vi "Ball Carrying Logic.vi"(0 "Backwards Trigger":dbl, 1 "Had Ball Before?":bool, 3 "Rollers Active? in":bool, 4 "Safty Frist Angle":dbl, 5 "Warmup Initiation":bool, 6 "Fire from Load Delay":i32, 7 "Intake Angle":dbl, 10 "Angle in":dbl, 11 "Intake at Dangerous Height?":bool, 12 "Roll Backward Delay":u32, 13 "Ball Loaded? in":bool) -> (14 "Rollers Active? out":bool, 15 "Angle out":dbl, 17 "Trigger Out":dbl, 18 "Ball Loaded? out":bool)   [LabVIEW 2015]
uses:
  Common Code/Change Detect Boolean.vi
  <vilib>/Rock Robotics/WPI/DriverStation/WPI_DriverStationRobotMode2.ctl
panel:
  in  "Safty Frist?":bool
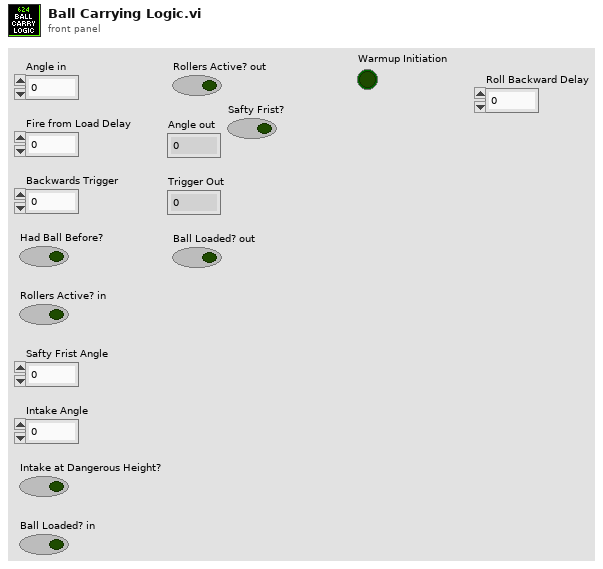
[diagram p1: front panel]
types:
  T1 = typedef "WPI_DriverStationRobotMode2.ctl" = enum16{"Autonomous Disabled", "Autonomous Enabled", "Teleop Disabled", "Teleop Enabled", "Disconnected", "Finish", "Test Disabled", "Test Enabled", "Emergency Stopped"}
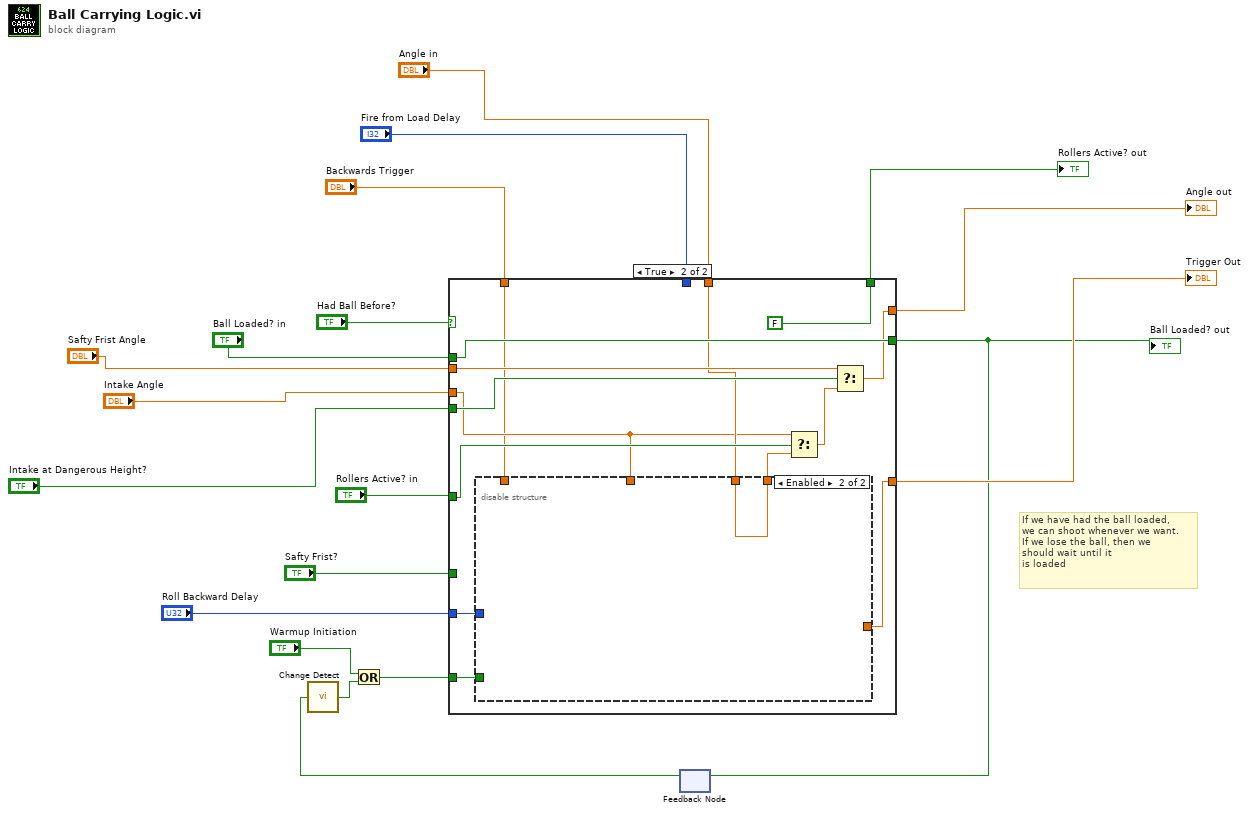
[diagram p0: block diagram]
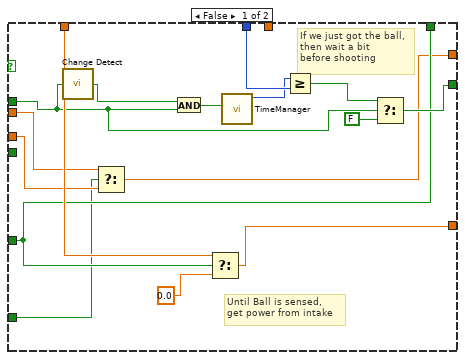
[diagram p2: hidden frame]
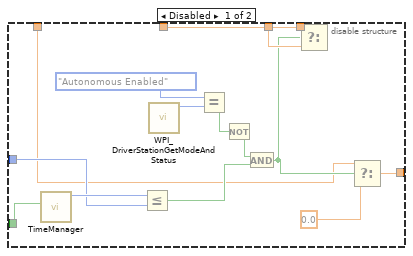
[diagram p3: hidden frame]
diagram:
  # "If we have had the ball loaded, \nwe can shoot whenever we want.\nIf we lose the ball, then we \nshould wait until it\nis loaded"
  n1 = feedback #1() -> (w3:bool)  [unwired: 1 in]
  n2 = call-poly "Change Detect.vi"("In"=w3) -> ("Changed?"=w2:bool)
  n3 = Or(x="Warmup Initiation", y=w2) -> (x .or. y?=w4:bool)
  n4 = case shown="True" "Had Ball Before?" {
    tunnel: "Fire from Load Delay" -> [w35 _]
    tunnel: "Ball Loaded? in" -> [w27 w49]
    tunnel: [w25 w49] -> w6
    tunnel: [w34 w41] -> w13
    tunnel: "Rollers Active? in" -> [w24 w44]
    tunnel: "Backwards Trigger" -> [w33 w36]
    tunnel: [w24 FALSE] -> w12
    tunnel: "Angle in" -> [_ w39]
    tunnel: [w21 w46] -> w15
    tunnel: "Intake Angle" -> [w23 w37]
    tunnel: "Intake at Dangerous Height?" -> [_ w45]
    tunnel: "Safty Frist Angle" -> [w22 w47]
    tunnel: "Safty Frist?" -> [w20 _]
    tunnel: w4 -> [_ w42]
    tunnel: "Roll Backward Delay" -> [_ w40]
    frame False {
      # "If we just got the ball,\nthen wait a bit\nbefore shooting"
      # "Until Ball is sensed,\nget power from intake"
      n5 = call-poly "Change Detect.vi"("In"=w27) -> ("Changed?"=w31:bool)
      n6 = Select(t=w22, s=w20, f=w23) -> (s? t:f=w21:dbl)
      n7 = And(x=w31, y=w27) -> (x .and. y?=w30:bool)
      n8 = Select(t=w33, s=w24, f=0.0 ("t")) -> (s? t:f=w34:dbl)
      n9 = call "TimeManager.vi"("Reset?"=w30) -> ("Time Since Reset"=w29:u32)  [unwired: 9 in, 1 out]
      n10 = Greater Or Equal?(x=w29, y=w35) -> (x >= y?=w28:bool)
      n11 = Select(t=w28, s=w27, f=FALSE) -> (s? t:f=w25:bool)
    }
    frame True {
      n12 = disable-structure shown="Enabled" {
        disable-tunnel: w42 -> [w64 _]
        disable-tunnel: [w62 _] -> w41
        disable-tunnel: w40 -> [w61 _]
        disable-tunnel: w39 -> [w60 w65]
        disable-tunnel: [w59 w65] -> w38
        disable-tunnel: w37 -> [w58 _]
        disable-tunnel: w36 -> [w51 _]
        frame Disabled {
          n13 = call "TimeManager.vi"("Reset?"=w64) -> ("Time Since Reset"=w63:u32)  [unwired: 9 in, 1 out]
          n14 = Less Or Equal?(x=w63, y=w61) -> (x <= y?=w53:bool)
          n15 = call <vilib>:"WPI_DriverStationGetModeAndStatus.vi"() -> ("Robot Mode"=w56:T1)  [unwired: 10 in, 1 out]
          n16 = Equal?(x=WPI_DriverStationRobotMode2."Autonomous Enabled", y=w56) -> (x = y?=w55:bool)
          n17 = Not(x=w55) -> (.not. x?=w54:bool)
          n18 = And(x=w54, y=w53) -> (x .and. y?=w52:bool)
          n19 = Select(t=w58, s=w52, f=w60) -> (s? t:f=w59:dbl)
          n20 = Select(t=w51, s=w52, f=0.0) -> (s? t:f=w62:dbl)
        }
        frame Enabled {
        }
      }
      n21 = Select(t=w37, s=w44, f=w38) -> (s? t:f=w43:dbl)
      n22 = Select(t=w47, s=w45, f=w43) -> (s? t:f=w46:dbl)
    }
  }
  "Angle out" <- w15
  "Trigger Out" <- w13
  "Rollers Active? out" <- w12
  "Ball Loaded? out" <- w6
  n23 = feedback-in #1(w6) -> ()
